vi "getReturn_NumpyArray2d_Bool.vi"(8 "error in (no error)":errorcluster, 9 "return list in":T1[](array[typedef]), 11 "LabVIEW-Python-Interface in":refnum<class "PyLVi.lvclass">) -> (0 "error out":errorcluster, 1 "return list out":T1[](array[typedef]), 2 "data out":bool[][](array[boolean]), 3 "LabVIEW-Python-Interface out":refnum<class "PyLVi.lvclass">)   [LabVIEW 2016, in "PyLVi.lvlib" / "PyLVi.lvclass"]
uses:
  PyLVi.lvclass
  Controls/ArgumentStructure.ctl
  Controls/DescriptorStructure.ctl
  Controls/ArgumentType.ctl
  Controls/DataType.ctl
panel:
  out "data string":string
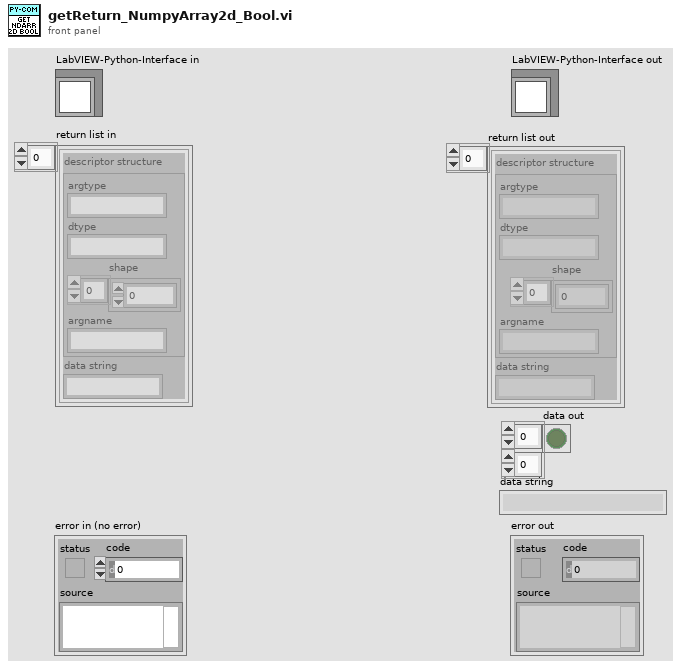
[diagram p1: front panel]
types:
  T1 = typedef "PyLVi.lvlib/PyLVi.lvclass/ArgumentStructure.ctl" = cluster{"descriptor structure":T2, "data string":string}
  T2 = typedef "PyLVi.lvlib/PyLVi.lvclass/DescriptorStructure.ctl" = cluster{"argtype":string, "dtype":string, "shape":u32[], "argname":string}
  T3 = enum16{"big-endian, network order", "native, host order", "little-endian"}
  T4 = typedef "PyLVi.lvlib/PyLVi.lvclass/DataType.ctl" = enum16{"bool", "string", "int16", "int32", "float32", "float64", "complex128"}
  T5 = typedef "PyLVi.lvlib/PyLVi.lvclass/ArgumentType.ctl" = enum8{"bool", "numeric", "string", "dict", "ndarray", "ndarray2d"}
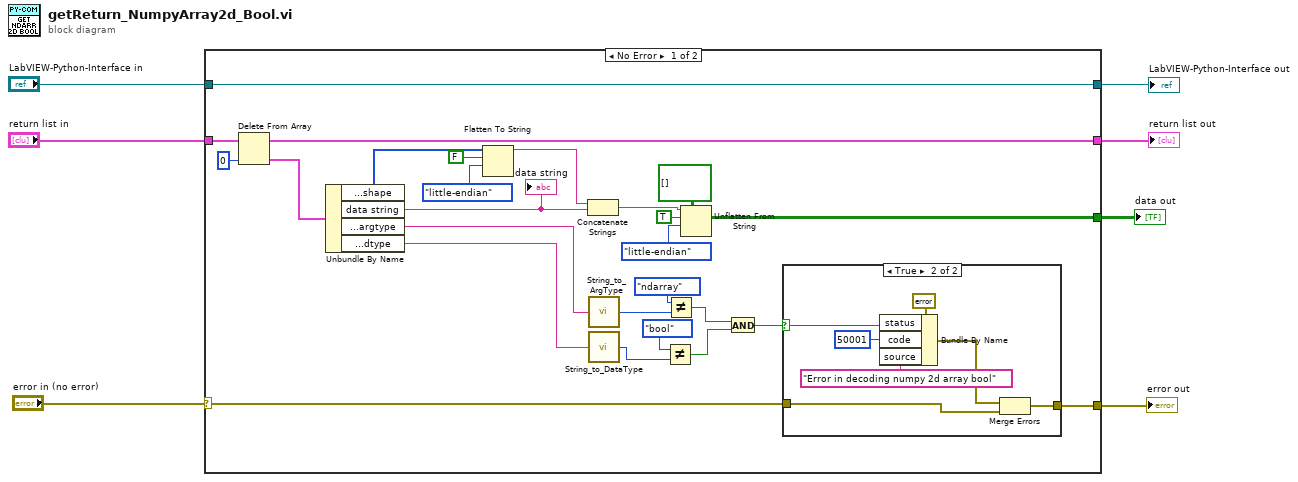
[diagram p0: block diagram]
diagram:
  n1 = case shown="No Error" "error in (no error)" {
    selector: "error in (no error)" -> [w9 w43]
    tunnel: [w10 w43] -> w2
    tunnel: [w18 w44] -> w5
    tunnel: "LabVIEW-Python-Interface in" -> [w18 w44]
    tunnel: "return list in" -> [w26 w42]
    tunnel: [w25 w42] -> w4
    tunnel: [w19 _] -> w1
    frame No Error {
      n2 = Delete From Array(array=w26, index=0) -> (deleted portion=w27:T1, array with subset deleted=w25:T1[])  [unwired: 1 in]
      n3 = Unbundle By Name(w27) -> ("descriptor structure.shape"=w15:u32[], "data string"=w14:string, "descriptor structure.argtype"=w24:string, "descriptor structure.dtype"=w23:string)
      "data string" <- w14
      n4 = Flatten To String(anything=w15, prepend array or string size? (T)=FALSE, byte order (0:big-endian, network order)=T3."little-endian") -> (data string=w13:string)  [unwired: 1 in, 2 out]
      n5 = Concatenate Strings(w13, w14) -> (w12:string)
      n6 = call "String_to_ArgType.vi"("arg type string"=w24) -> ("arg type"=w28:T5)  [unwired: 4 in]
      n7 = call "String_to_DataType.vi"("data type string"=w23) -> ("data type"=w30:T4)  [unwired: 4 in]
      n8 = Not Equal?(x=DataType."bool", y=w30) -> (x != y?=w33:bool)
      n9 = Not Equal?(x=ArgumentType."ndarray", y=w28) -> (x != y?=w32:bool)
      n10 = Unflatten From String(type=bool[][] [], binary string=w12, data includes array or string size? (T)=TRUE, byte order (0:big-endian, network order)=T3."little-endian") -> (value=w19:bool[][])  [unwired: 1 in, 2 out]
      n11 = And(x=w32, y=w33) -> (x .and. y?=w11:bool)
      n12 = case shown="True" w11 {
        selector: w11 -> [_ w38]
        tunnel: [w34 w37] -> w10
        tunnel: w9 -> [w34 w35]
        frame False {
        }
        frame True {
          n13 = Bundle By Name(cluster=errorcluster {"status"=FALSE, "code"=0, "source"=""} ("error constant"), "status"=w38, "code"=50001, "source"="Error in decoding numpy 2d array bool") -> (w36:errorcluster)
          n14 = Merge Errors(w36, w35) -> (w37:errorcluster)
        }
      }
    }
    frame Error {
    }
  }
  "error out" <- w2
  "LabVIEW-Python-Interface out" <- w5
  "return list out" <- w4
  "data out" <- w1
